vi "Delay, Seconds.vi"(4 "enable (T)":bool=TRUE, 5 "error in":errorcluster, 8 "delay":dbl[unit]=0.1 caption="Delay" format="%_3g") -> (0 "error out":errorcluster {"code" format="%.0x"}, 3 "ms timer value":u32)   [LabVIEW 2020]
doc: "Delay, if no error and enabled."
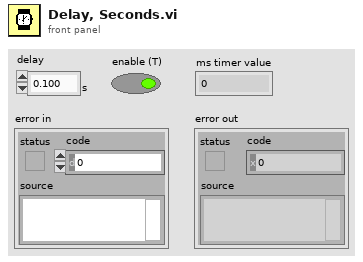
[diagram p1: front panel]
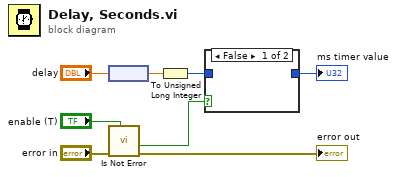
[diagram p0: block diagram]
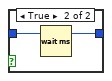
[diagram p2: hidden frame]
diagram:
  n1 = node("delay") -> (w7:dbl)
  n2 = call "Is Not Error.vi"("enable (T)"="enable (T)", "error in"="error in") -> ("error out"=→"error out":errorcluster, "ready"=w2:bool)  [unwired: 4 in, 1 out]
  n3 = To Unsigned Long Integer(number=w7) -> (unsigned 32bit integer=w6:u32)
  n4 = case shown="False" w2 {
    tunnel: w6 -> [_ w10]
    tunnel: [_ w9] -> w5
    frame False {
    }
    frame True {
      n5 = Wait (ms)(milliseconds to wait=w10) -> (millisecond timer value=w9:u32)
    }
  }
  "ms timer value" <- w5
